vi "Get SubPanel Reference.vi"(8 "error in (no error)":errorcluster, 11 "Dumb Plugin in":refnum<class "Dumb Plugin.lvclass">) -> (0 "error out":errorcluster, 2 "VI Ref":refnum<vi>, 3 "Dumb Plugin out":refnum<class "Dumb Plugin.lvclass">)   [LabVIEW 2011, in "Dumb Plugin.lvclass"]
uses:
  Dumb Plugin.lvclass
  Generate Waveform.vi
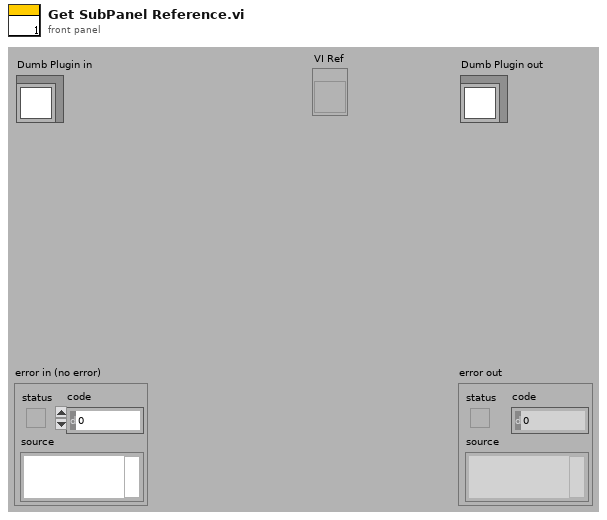
[diagram p1: front panel]
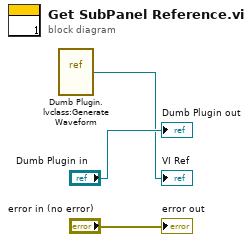
[diagram p0: block diagram]
diagram:
  n1 = vi-ref "Dumb Plugin.lvclass:Generate Waveform.vi"() -> (→"VI Ref":refnum<vi>)
  "error out" <- "error in (no error)"
  "Dumb Plugin out" <- "Dumb Plugin in"
